vi "Error Handler.vi"(8 "Engine Error":errorcluster, 11 "Component Info In":T1) -> (0 "Engine Errors":errorcluster, 1 "Safe State":bool, 3 "Component Info Out":T1)   [LabVIEW 2013, in "Standard Engine Runtime.lvclass"]
uses:
  Standard Engine Runtime.lvclass
  Module Execution Info.ctl
  <vilib>/NI/Tag Bus Module Framework/runtime/TBM module execution interface.lvclass
  Data Table with Transfer Spec.ctl
  <vilib>/NI/Tag Bus/table/data table.ctl
  <vilib>/NI/Tag Bus/table/transfer specification.ctl
  <vilib>/NI/Tag Bus/tag/Data Type.ctl
  Configuration/Module Decimation.ctl
  Configuration/Module Error Configuration.ctl
  Configuration/Error Actions By Category.ctl
  <vilib>/NI/Tag Bus Module Framework/runtime/error classification.ctl
  Configuration/Error Actions.ctl
  Configuration/Standard Engine Configuration.lvclass
  <vilib>/NI/Tag Bus/tag/tag descriptor.lvclass
  <vilib>/NI/Tag Bus/table/data table.lvlib
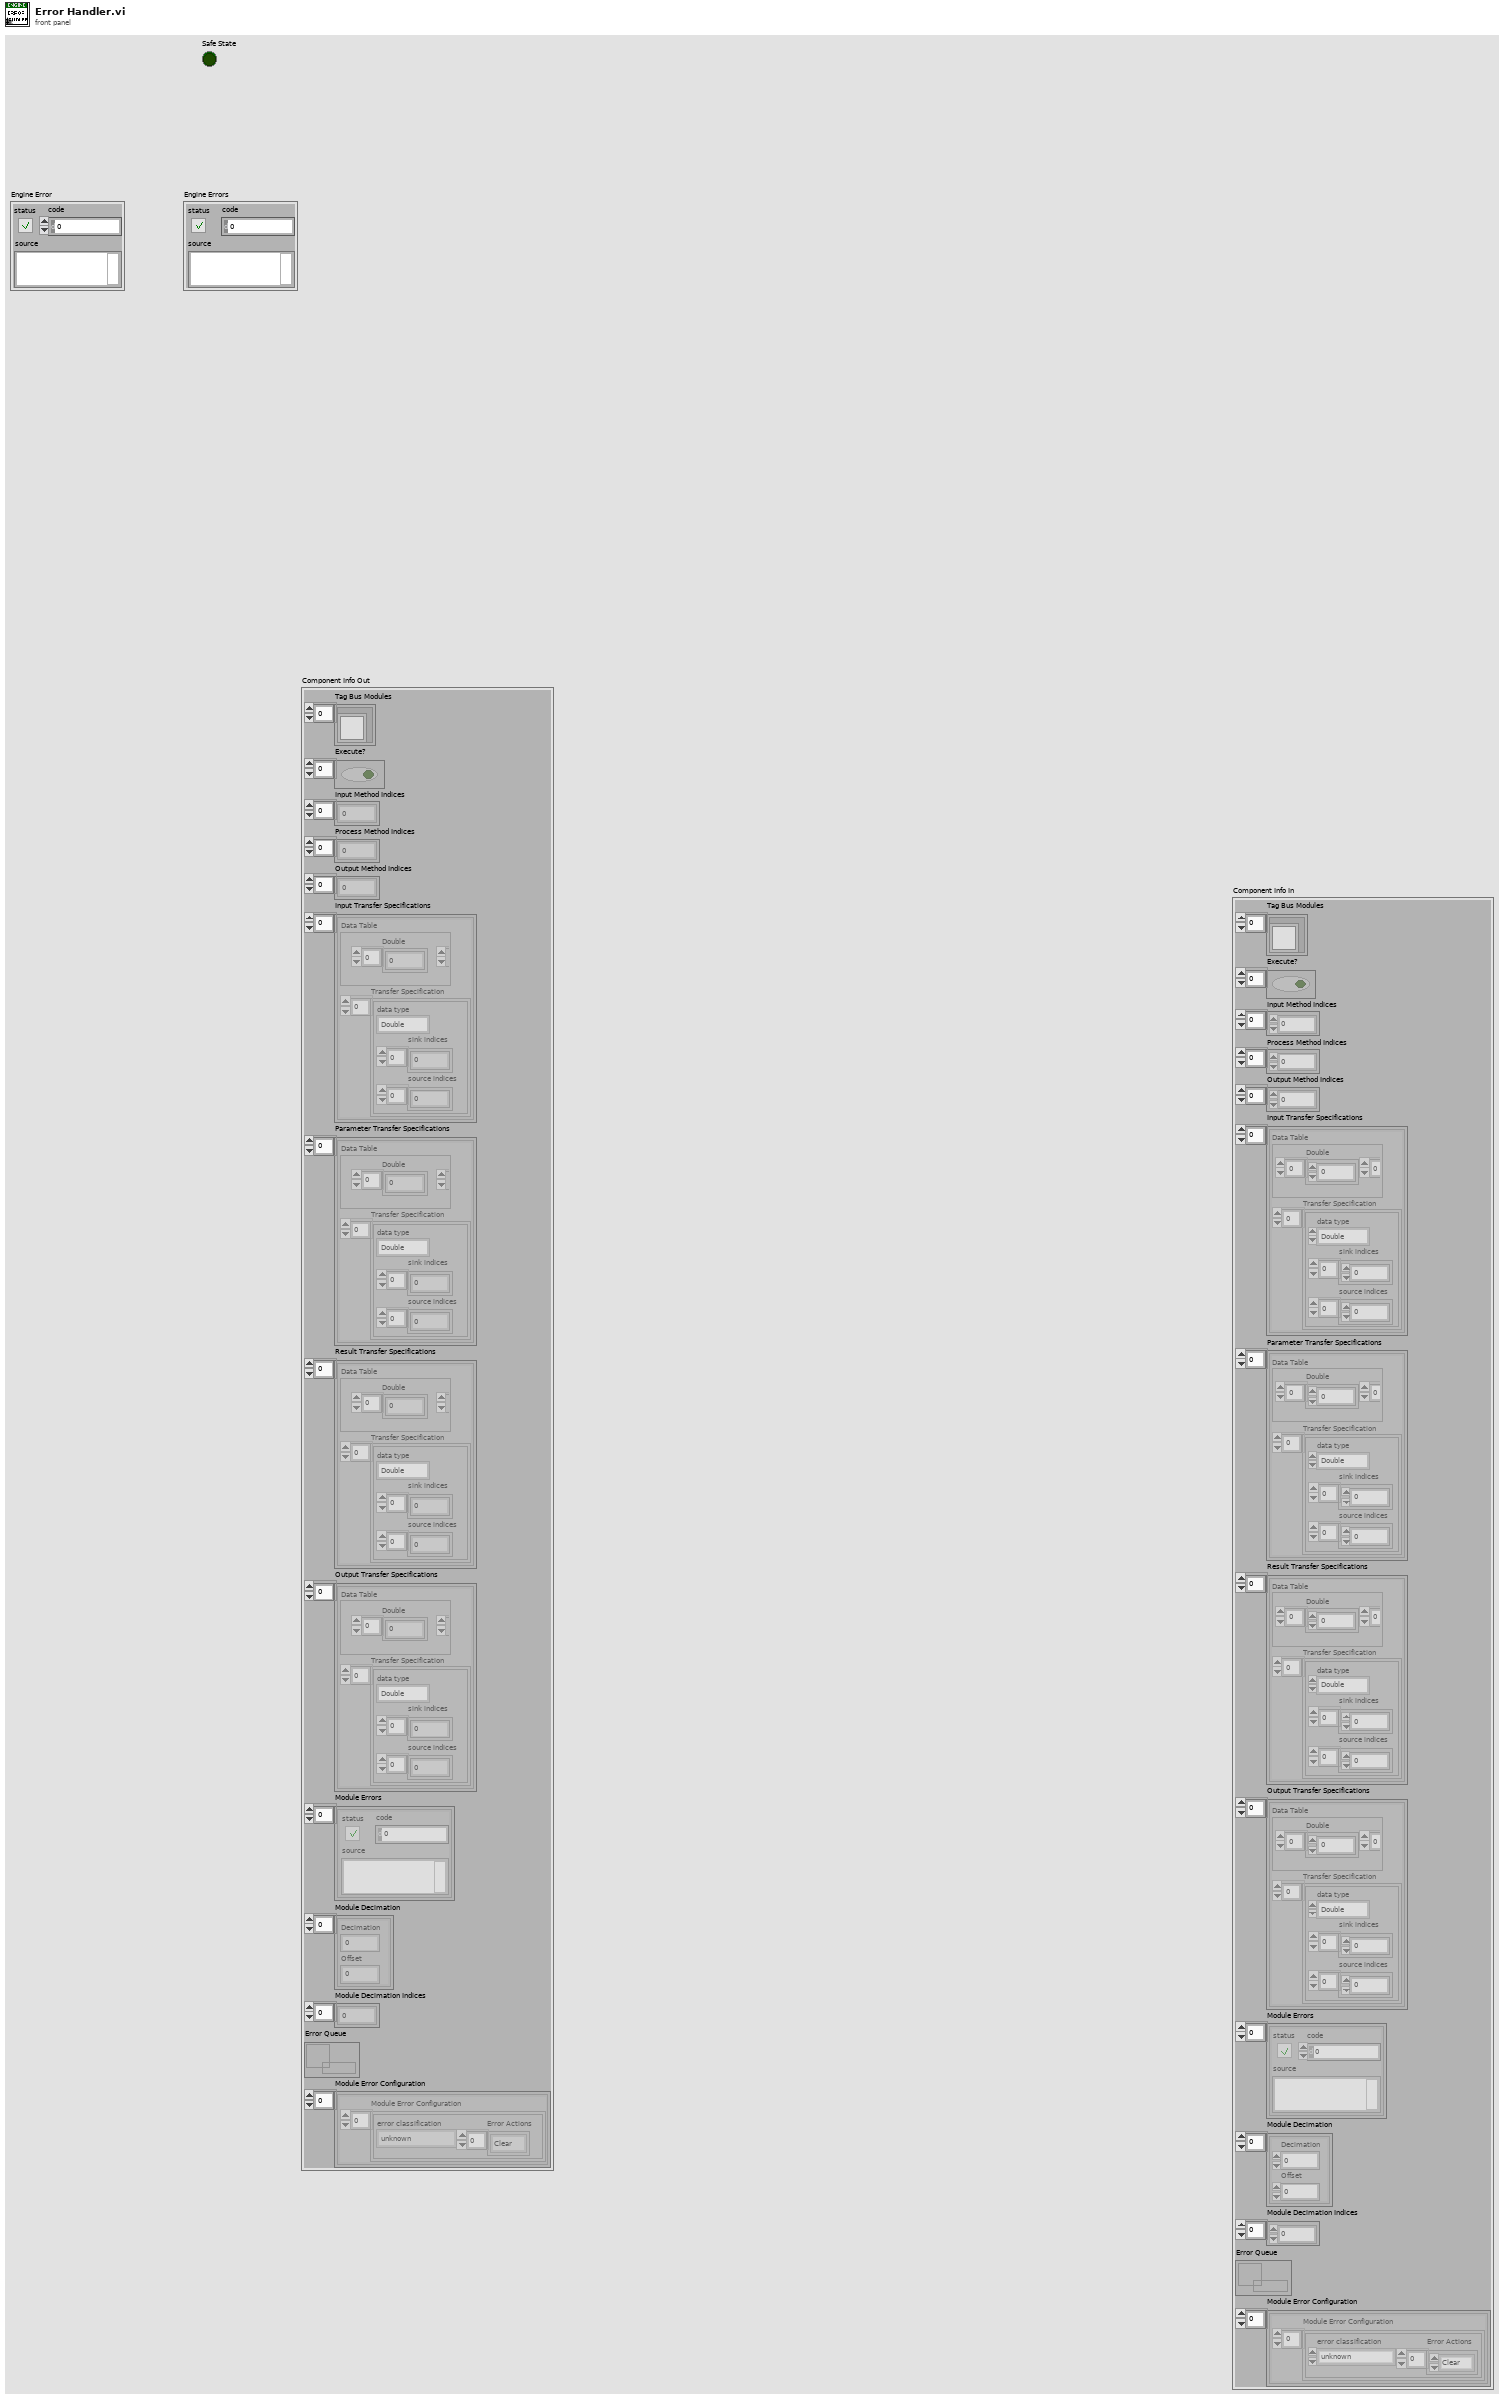
[diagram p1: front panel]
types:
  T1 = typedef "Standard Engine Runtime.lvclass/Module Execution Info.ctl" = cluster{"Tag Bus Modules":refnum<class "TBM module execution interface.lvclass">[], "Execute?":bool[], "Input Method Indices":i32[], "Process Method Indices":i32[], "Output Method Indices":i32[], "Input Transfer Specifications":T2[], "Parameter Transfer Specifications":T2[], "Result Transfer Specifications":T2[], "Output Transfer Specifications":T2[], "Module Errors":errorcluster[], "Module Decimation":T6[], "Module Decimation Indices":i32[], "Error Queue":refnum<queue>, "Module Error Configuration":T7[]}
  T2 = typedef "Standard Engine Runtime.lvclass/Data Table with Transfer Spec.ctl" = cluster{"Data Table":T3, "Transfer Specification":T4[]}
  T3 = typedef "tag bus.lvlib/data table.lvlib/data table.ctl" = cluster{"Double":dbl[], "Single":sgl[], "I64":i64[], "I32":i32[], "I16":i16[], "I8":i8[], "U64":u64[], "U32":u32[], "U16":u16[], "U8":u8[], "Boolean":bool[], "String":string[], "Array of Double":cluster{"DBL Array":dbl[]}[], "Array of Single":cluster{"SGL Array":sgl[]}[], "Array of I64":cluster{"I64 Array":i64[]}[], "Array of I32":cluster{"I32 Array":i32[]}[], "Array of I16":cluster{"I16 Array":i16[]}[], "Array of I8":cluster{"I8 Array":i8[]}[], "Array of U64":cluster{"U64 Array":u64[]}[], "Array of U32":cluster{"U32 Array":u32[]}[], "Array of U16":cluster{"U16 Array":u16[]}[], "Array of U8":cluster{"U8 Array":u8[]}[], "Array of Boolean":cluster{"Boolean Array":bool[]}[], "Array of String":cluster{"String Array":string[]}[]}
  T4 = typedef "tag bus.lvlib/data table.lvlib/transfer specification.ctl" = cluster{"data type":T5, "sink indices":i32[], "source indices":i32[]}
  T5 = typedef "tag bus.lvlib/tag descriptor.lvclass/Data Type.ctl" = enum16{"Double", "Single", "I64", "I32", "I16", "I8", "U64", "U32", "U16", "U8", "Boolean", "String", "Array of Double", "Array of Single", "Array of I64", "Array of I32", "Array of I16", "Array of I8", "Array of U64", "Array of U32", "Array of U16", "Array of U8", "Array of Boolean", "Array of String"}
  T6 = typedef "Standard Engine Configuration.lvclass/Module Decimation.ctl" = cluster{"Decimation":u16, "Offset":u16}
  T7 = typedef "Standard Engine Configuration.lvclass/Module Error Configuration.ctl" = cluster{"Module Error Configuration":T8[]}
  T8 = typedef "Standard Engine Configuration.lvclass/Error Actions By Category.ctl" = cluster{"error classification":T9, "Error Actions":T10[]}
  T9 = typedef "TBM module execution interface.lvclass/error classification.ctl" = enum16{"unknown", "none", "trivial", "recoverable", "critical"}
  T10 = typedef "Standard Engine Configuration.lvclass/Error Actions.ctl" = enum16{"Clear", "Notify", "Stop Component", "Stop Engine", "Safe State", "Attempt Recovery"}
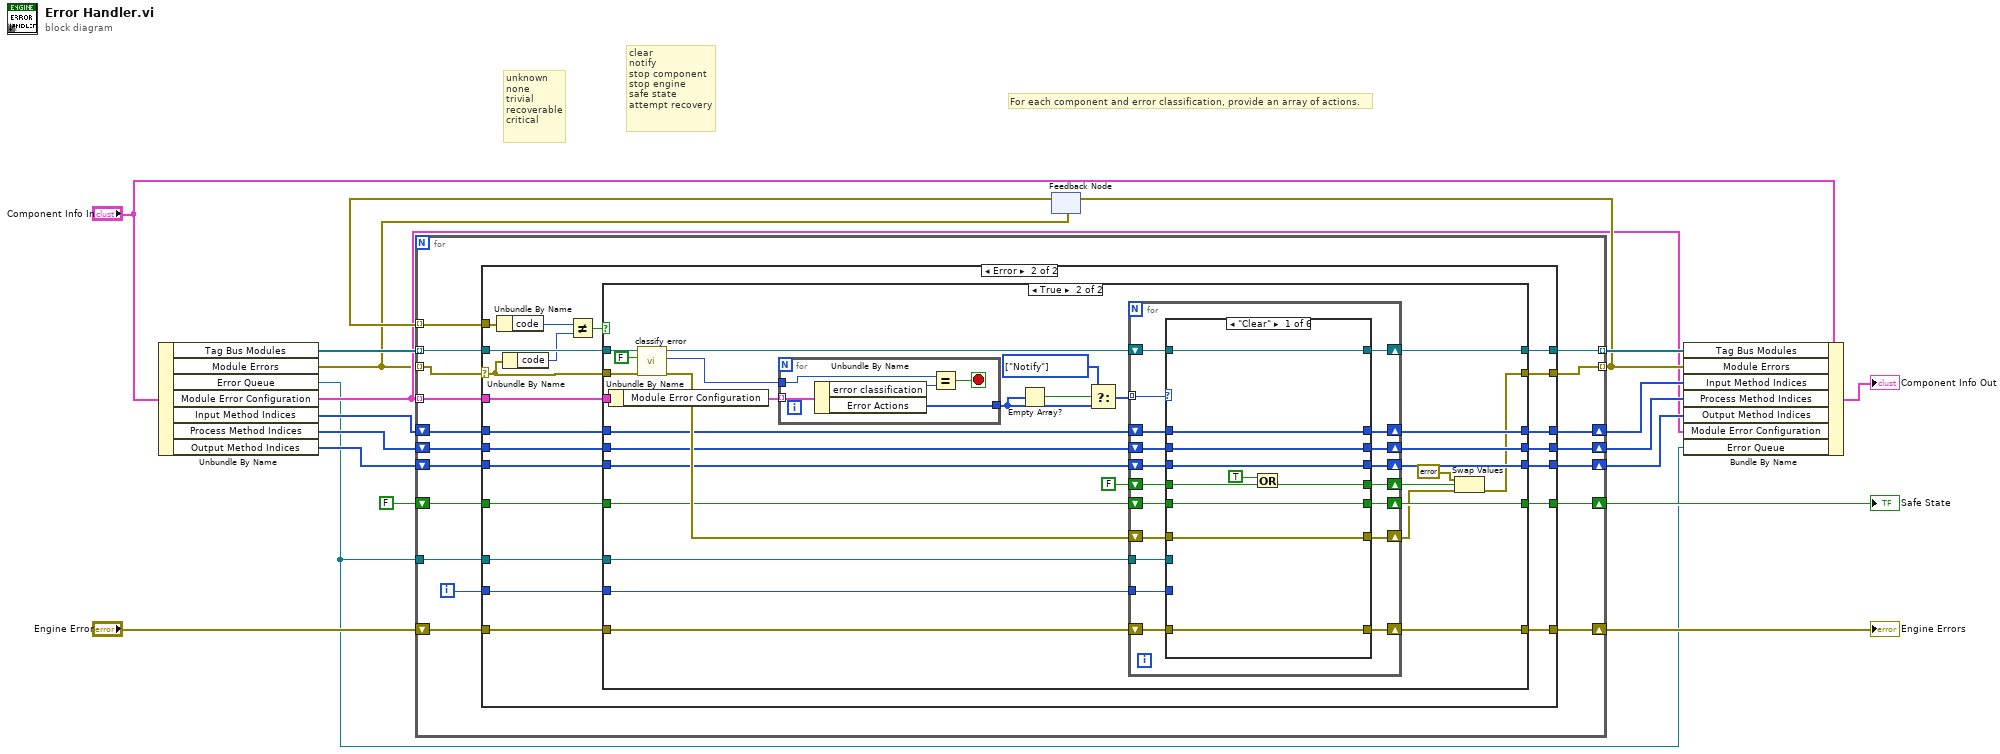
[diagram p0: block diagram]
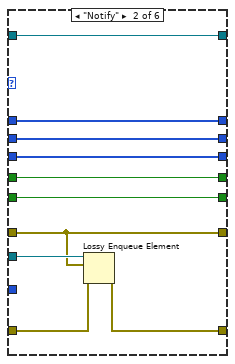
[diagram p4: hidden frame]
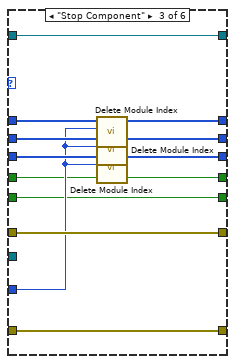
[diagram p5: hidden frame]
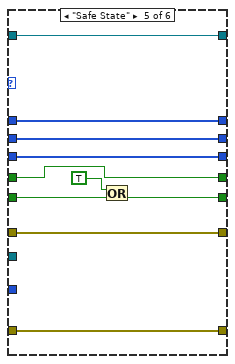
[diagram p7: hidden frame]
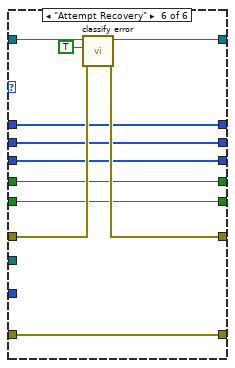
[diagram p8: hidden frame]
diagram:
  # "clear\nnotify\nstop component\nstop engine\nsafe state\nattempt recovery"
  # "unknown\nnone\ntrivial\nrecoverable\ncritical"
  # "For each component and error classification, provide an array of actions."
  n1 = Unbundle By Name("Component Info In") -> ("Tag Bus Modules"=w17:refnum<class "TBM module execution interface.lvclass">[], "Module Errors"=w1:errorcluster[], "Error Queue"=w2:refnum<queue>, "Module Error Configuration"=w3:T7[], "Input Method Indices"=w13:i32[], "Process Method Indices"=w12:i32[], "Output Method Indices"=w11:i32[])
  n2 = feedback #1(w1) -> (w6:errorcluster[])
  n3 = for {
    tunnel: w1 -> [w31] mode=indexing
    tunnel: [w35] -> w7 mode=indexing
    tunnel: [w34] -> w15 mode=indexing
    tunnel: w17 -> [w32] mode=indexing
    tunnel: w3 -> [w33] mode=indexing
    shift-right: [w36] -> w19
    shift-left: "Engine Error" -> [w37]
    tunnel: w2 -> [w30]
    shift-right: [w26] -> w10
    shift-left: w13 -> [w29]
    shift-right: [w25] -> w9
    shift-left: w12 -> [w28]
    shift-right: [w24] -> w8
    shift-left: w11 -> [w27]
    tunnel: w6 -> [w22] mode=indexing
    shift-right: [w21] -> w4
    shift-left: FALSE -> [w20]
    i -> [w23]
    n4 = case shown="Error" w31 {
      selector: w31 -> [w42 w50]
      tunnel: w37 -> [w44 w62]
      tunnel: [w44 w61] -> w36
      tunnel: [w42 w64] -> w35
      tunnel: [w43 w63] -> w34
      tunnel: w32 -> [w43 w65]
      tunnel: w33 -> [_ w52]
      tunnel: w30 -> [_ w60]
      tunnel: w29 -> [w41 w59]
      tunnel: w28 -> [w40 w58]
      tunnel: w27 -> [w39 w57]
      tunnel: [w41 w56] -> w26
      tunnel: [w40 w55] -> w25
      tunnel: [w39 w54] -> w24
      tunnel: w23 -> [_ w53]
      tunnel: w22 -> [_ w51]
      tunnel: [w38 w45] -> w21
      tunnel: w20 -> [w38 w46]
      frame No Error {
      }
      frame Error {
        n5 = Unbundle By Name(w51) -> ("code"=w49:i32)
        n6 = Unbundle By Name(w50) -> ("code"=w48:i32)
        n7 = Not Equal?(x=w49, y=w48) -> (x != y?=w47:bool)
        n8 = case shown="True" w47 {
          tunnel: w65 -> [w72 w101]
          tunnel: [w71 w74] -> w64
          tunnel: [w72 w98] -> w63
          tunnel: w62 -> [w67 w97]
          tunnel: [w67 w96] -> w61
          tunnel: w60 -> [_ w95]
          tunnel: w59 -> [w70 w94]
          tunnel: w58 -> [w69 w93]
          tunnel: w57 -> [w68 w92]
          tunnel: [w70 w91] -> w56
          tunnel: [w69 w90] -> w55
          tunnel: [w68 w89] -> w54
          tunnel: w53 -> [_ w88]
          tunnel: w52 -> [_ w87]
          tunnel: w50 -> [w71 w80]
          tunnel: w46 -> [w66 w79]
          tunnel: [w66 w78] -> w45
          frame False {
          }
          frame True {
            w81 = T10[] [enum."Notify"] items=["Clear", "Notify", "Stop Component", "Stop Engine", "Safe State", "Attempt Recovery"] ("t")
            n9 = Unbundle By Name(w87) -> ("Module Error Configuration"=w86:T8[])
            n10 = call-dynamic "classify error.vi"("error to classify"=w80, "attempt recovery?"=FALSE, "module in"=w101) -> ("classified error"=w100:errorcluster, "error classification"=w85:T9, "module out"=w99:refnum<class "TBM module execution interface.lvclass">)  [unwired: 6 in]
            n11 = for {
              tunnel: w86 -> [w107] mode=indexing
              tunnel: w85 -> [w106]
              tunnel: [w103] -> w83
              stop <- w104 stop-if-true
              n12 = Unbundle By Name(w107) -> ("error classification"=w105:T9, "Error Actions"=w103:T10[])
              n13 = Equal?(x=w106, y=w105) -> (x = y?=w104:bool)
            }
            n14 = Empty Array?(array=w83) -> (empty?=w84:bool)
            n15 = Select(t=w81, s=w84, f=w83) -> (s? t:f=w82:T10[])
            n16 = for {
              tunnel: w82 -> [w126] mode=indexing
              shift-right: [w125] -> w75
              shift-left: w100 -> [w124]
              shift-right: [w120] -> w96
              shift-left: w97 -> [w121]
              shift-right: [w123] -> w98
              shift-left: w99 -> [w122]
              tunnel: w95 -> [w119]
              shift-right: [w117] -> w91
              shift-left: w94 -> [w118]
              shift-right: [w115] -> w90
              shift-left: w93 -> [w116]
              shift-right: [w113] -> w89
              shift-left: w92 -> [w114]
              tunnel: w88 -> [w112]
              shift-right: [w110] -> w78
              shift-left: w79 -> [w111]
              shift-right: [w109] -> w76
              shift-left: FALSE -> [w108]
              n17 = case shown="\"Clear\"" w126 {
                tunnel: [w130 w139 w158 w164 w174 w182] -> w125
                tunnel: w124 -> [w130 w139 w158 w164 w174 w183]
                tunnel: [w136 w146 w157 w165 w175 w185] -> w123
                tunnel: w122 -> [w136 w146 w157 w165 w175 w186]
                tunnel: w121 -> [w135 w140 w156 _ w170 w181]
                tunnel: [w135 w144 w156 w164 w170 w181] -> w120
                tunnel: w119 -> [_ w145 _ _ _ _]
                tunnel: w118 -> [w134 w143 w155 w163 w173 w180]
                tunnel: [w134 w143 w154 w163 w173 w180] -> w117
                tunnel: w116 -> [w133 w142 w153 w162 w172 w179]
                tunnel: [w133 w142 w151 w162 w172 w179] -> w115
                tunnel: w114 -> [w132 w141 w152 w161 w171 w178]
                tunnel: [w132 w141 w150 w161 w171 w178] -> w113
                tunnel: w112 -> [_ _ w149 _ _ _]
                tunnel: w111 -> [w131 w138 w148 w160 w169 w177]
                tunnel: [w131 w138 w148 w160 w168 w177] -> w110
                tunnel: [w128 w137 w147 w159 w166 w176] -> w109
                tunnel: w108 -> [w129 w137 w147 w159 w166 w176]
                frame "Clear" {
                  n18 = Or(x=TRUE, y=w129) -> (x .or. y?=w128:bool)
                }
                frame "Notify" {
                  n19 = Lossy Enqueue Element(queue=w145, element=w139, error in (no error)=w140) -> (error out=w144:errorcluster)  [unwired: 3 out]
                }
                frame "Stop Component" {
                  n20 = call "Delete Module Index.vi"("Index"=w149, "Module Indices"=w155) -> ("Module Indices"=w154:i32[])  [unwired: 9 in]
                  n21 = call "Delete Module Index.vi"("Index"=w149, "Module Indices"=w153) -> ("Module Indices"=w151:i32[])  [unwired: 9 in]
                  n22 = call "Delete Module Index.vi"("Index"=w149, "Module Indices"=w152) -> ("Module Indices"=w150:i32[])  [unwired: 9 in]
                }
                frame "Stop Engine" {
                  # "Passing an engine error out stops the engine."
                }
                frame "Safe State" {
                  n23 = Or(x=TRUE ("Stop Engine"), y=w169) -> (x .or. y?=w168:bool)
                }
                frame "Attempt Recovery" {
                  n24 = call-dynamic "classify error.vi"("error to classify"=w183, "attempt recovery?"=TRUE, "module in"=w186) -> ("classified error"=w182:errorcluster, "module out"=w185:refnum<class "TBM module execution interface.lvclass">)  [unwired: 6 in, 1 out]
                }
              }
            }
            n25 = Swap Values(12:errorcluster {"status"=FALSE, "code"=0, "source"=""} ("classified error"), 13:w76, 14:w75) -> (3:w74:errorcluster)  [unwired: 1 out]
          }
        }
      }
    }
  }
  "Engine Errors" <- w19
  "Safe State" <- w4
  n26 = feedback-in #1(w7) -> ()
  n27 = Bundle By Name(cluster="Component Info In", "Tag Bus Modules"=w15, "Module Errors"=w7, "Input Method Indices"=w10, "Process Method Indices"=w9, "Output Method Indices"=w8, "Module Error Configuration"=w3, "Error Queue"=w2) -> (→"Component Info Out":T1)
